vi "isNull.vi"(11 "LQIdentity In":refnum<class "LQIdentity.lvclass">) -> (2 "Is Null?":bool, 3 "LQIdentity Out":refnum<class "LQIdentity.lvclass">)   [LabVIEW 2014, in "LQ Core.lvlib" / "LQIdentity.lvclass"]
uses:
  LQIdentity.lvclass
  LQIdentity.lvclass/LQIdentity.ctl
panel:
  # "Copyright (c) 2016 Sze Howe Koh\n\nThis Source Code Form is subject to the terms of the Mozilla Public\nLicense, v. 2.0. If a copy of the MPL was not distributed with this\nfile, You can obtain one at http://mozilla.org/MPL/2.0/."
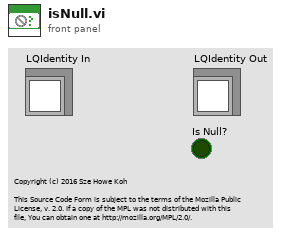
[diagram p1: front panel]
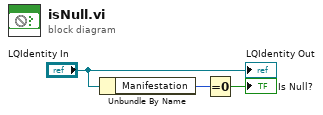
[diagram p0: block diagram]
diagram:
  n1 = Unbundle By Name("LQIdentity In") -> ("Manifestation"=w2:u64)
  n2 = Equal To 0?(x=w2) -> (x = 0?=→"Is Null?":bool)
  "LQIdentity Out" <- "LQIdentity In"
